vi "seconds2time.vi"(11 "seconds":dbl) -> (3 "HH:MM:SS":string)   [LabVIEW 2018]
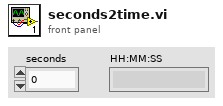
[diagram p1: front panel]
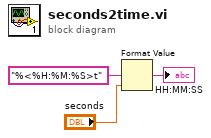
[diagram p0: block diagram]
diagram:
  n1 = Format Value(format string="%<%H:%M:%S>t", value (0)="seconds") -> (output string=→"HH:MM:SS":string)  [unwired: 1 in]
